vi "BRig_RT_comm_webdav_upload__checkData.vi"(8 "input_error":errorcluster, 10 "input_targetPath":string, 11 "input_hSession":T1) -> (0 "error out":errorcluster, 2 "output_checkData":bool, 3 "output_hSession":T1)   [LabVIEW 2014]
uses:
  <vilib>/WebDAVClient/Advanced/SessionHandle.ctl
  <vilib>/WebDAVClient/NI_WebDAV.lvlib
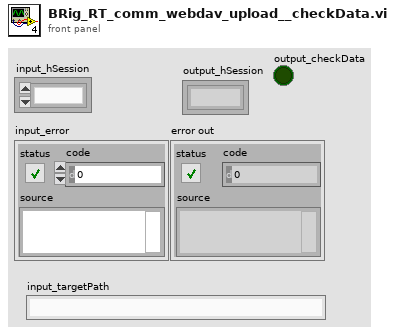
[diagram p1: front panel]
types:
  T1 = typedef "NI_WebDAV.lvlib/SessionHandle.ctl" = refnum<k1>
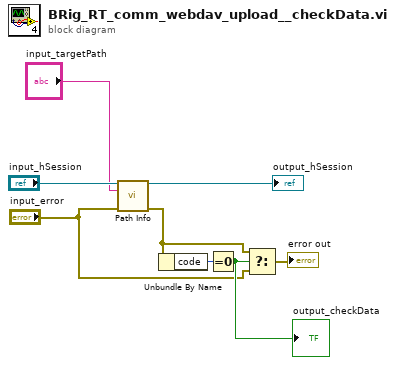
[diagram p0: block diagram]
diagram:
  n1 = call <vilib>:"Path Info.vi"("session handle"="input_hSession", "relative uri"="input_targetPath", "error in (no error)"="input_error") -> ("session handle out"=→"output_hSession":T1, "error out"=w4:errorcluster)  [unwired: 9 in, 2 out]
  n2 = Unbundle By Name(w4) -> ("code"=w7:i32)
  n3 = Equal To 0?(x=w7) -> (x = 0?=w5:bool)
  "output_checkData" <- w5
  n4 = Select(t=w4, s=w5, f="input_error") -> (s? t:f=→"error out":errorcluster)
